vi "TDMS Advanced Asynchronous Read Speed Test.vi"(7 "Debug":bool, 8 "Error In":errorcluster, 10 "Tree Selection":T1, 11 "TDMS Data Save":T2) -> (0 "Error Out":errorcluster, 1 "channel name(s) out":string[](array[string]), 2 "TDMS Data":T3, 3 "TDMS Data Save Output":T2)   [LabVIEW 2016]
doc: "This example demonstrates how to benchmark the streaming performance when you use the TDMS Advanced Asynchronous I/O functions to read data from a .tdms file. This VI measures the time it takes to continuously read data from a file and calculates the average data throughput in bytes/second."
uses:
  Refrigeration/RTS/Type Definitions/RTS TDMS Data.ctl
  Refrigeration/RTS/Type Definitions/RTS TDMS Filename Locations.ctl
  Refrigeration/RTS/Type Definitions/RTS Room Selector.ctl
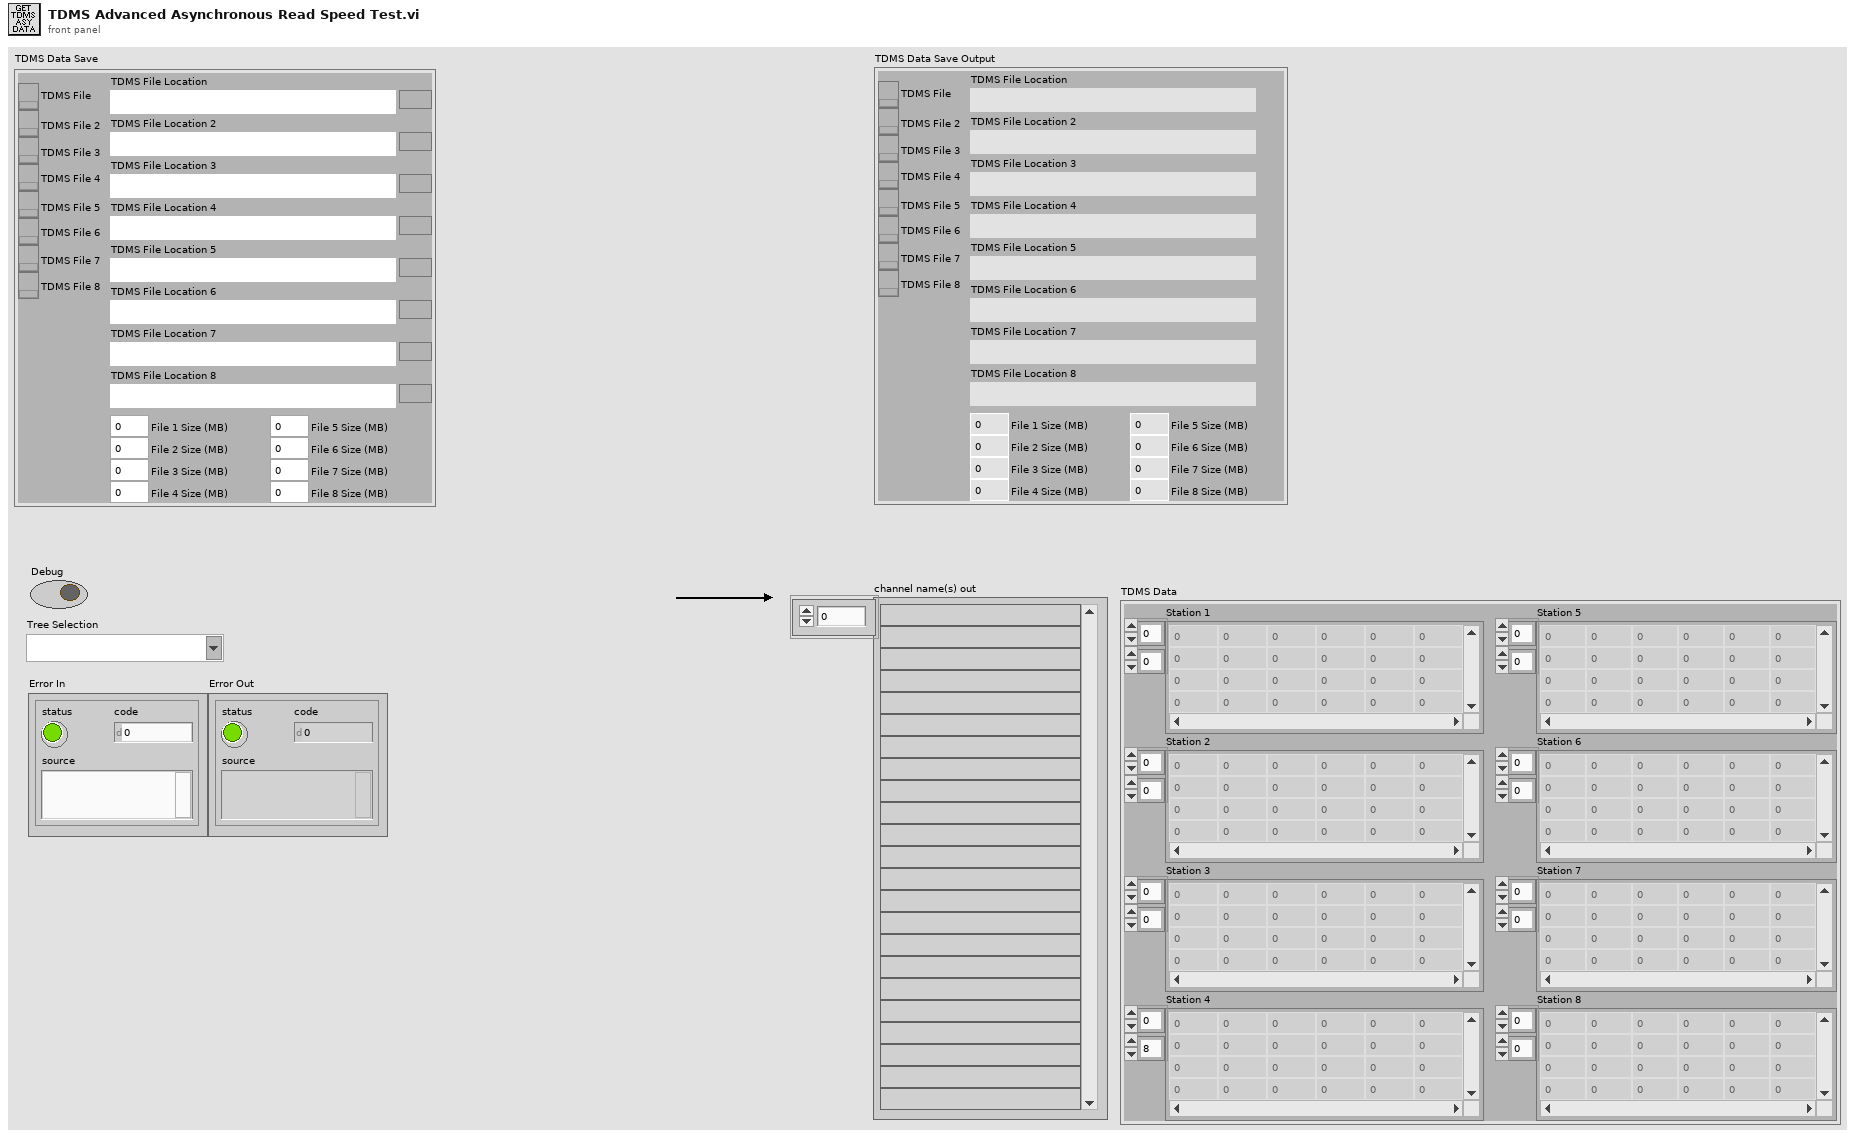
[diagram p1: front panel]
types:
  T1 = typedef "RTS Room Selector.ctl" = string
  T2 = typedef "RTS TDMS Filename Locations.ctl" = cluster{"TDMS File":refnum<k34>, "TDMS File Location":path, "TDMS File Location 2":path, "TDMS File Location 3":path, "TDMS File Location 4":path, "TDMS File Location 5":path, "TDMS File Location 6":path, "TDMS File Location 7":path, "TDMS File Location 8":path, "TDMS File 2":refnum<k34>, "TDMS File 3":refnum<k34>, "TDMS File 4":refnum<k34>, "TDMS File 5":refnum<k34>, "TDMS File 6":refnum<k34>, "TDMS File 7":refnum<k34>, "TDMS File 8":refnum<k34>, "File 1 Size (MB)":dbl, "File 2 Size (MB)":dbl, "File 3 Size (MB)":dbl, "File 4 Size (MB)":dbl, "File 5 Size (MB)":dbl, "File 6 Size (MB)":dbl, "File 7 Size (MB)":dbl, "File 8 Size (MB)":dbl}
  T3 = typedef "RTS TDMS Data.ctl" = cluster{"Station 1":dbl[][], "Station 2":dbl[][], "Station 3":dbl[][], "Station 4":dbl[][], "Station 5":dbl[][], "Station 6":dbl[][], "Station 7":dbl[][], "Station 8":dbl[][]}
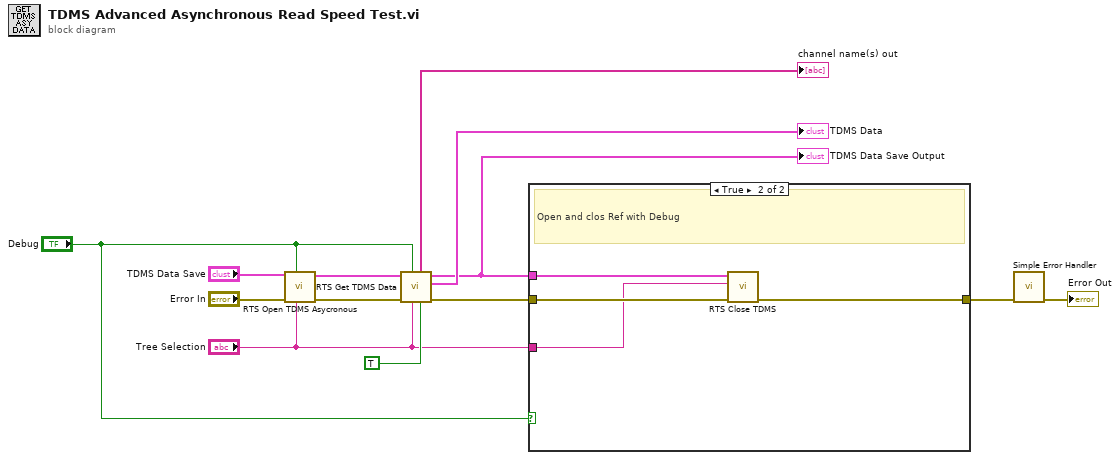
[diagram p0: block diagram]
diagram:
  n1 = call "RTS Open TDMS Asycronous.vi"("Tree Selection"="Tree Selection", "Debug"="Debug", "Error In"="Error In", "TDMS Data Save Input"="TDMS Data Save") -> ("Error Out"=w12:errorcluster, "TDMS Data Save Output"=w8:T2)  [unwired: 6 in]
  n2 = call "RTS Get TDMS Data.vi"("Read All?"=TRUE, "Tree Selection"="Tree Selection", "Debug"="Debug", "error in (no error)"=w12, "TDMS Data Save"=w8) -> ("error out"=w11:errorcluster, "TDMS Data Output"=→"TDMS Data":T3, "TDMS Data Save Output"=w2:T2, "channel name(s) out"=→"channel name(s) out":string[])  [unwired: 3 in]
  "TDMS Data Save Output" <- w2
  n3 = case shown="True" "Debug" {
    tunnel: [w14 w16] -> w13
    tunnel: w2 -> [_ w18]
    tunnel: w11 -> [w14 w17]
    tunnel: "Tree Selection" -> [_ w15]
    frame False {
      # "It takes time to open ref. So just leave it open when reading"
    }
    frame True {
      # "Open and clos Ref with Debug"
      n4 = call "RTS Close TDMS.vi"("Error In"=w17, "Tree Selection"=w15, "TDMS Data Save in"=w18) -> ("Error Out"=w16:errorcluster)  [unwired: 7 in, 1 out]
    }
  }
  n5 = call <vilib>:"Simple Error Handler.vi"("error in (no error)"=w13) -> ("error out"=→"Error Out":errorcluster)  [unwired: 1 in, 7 out]
